vi "VCI Read Board Info.vi"(8 "error in (no error)":errorcluster, 10 "DevIndex":u32, 11 "DevType":u32) -> (0 "error out":errorcluster, 2 "function return":u32, 3 "pInfo":T1)   [LabVIEW 2012, in "ControlCAN.lvlib"]
doc: "unsigned int WINAPI VCI_ReadBoardInfo(unsigned int DevType,unsigned int DevIndex,PVCI_BOARD_INFO pInfo);"
uses:
  ControlCAN.lvlib
  Ginkgo_Driver.dll
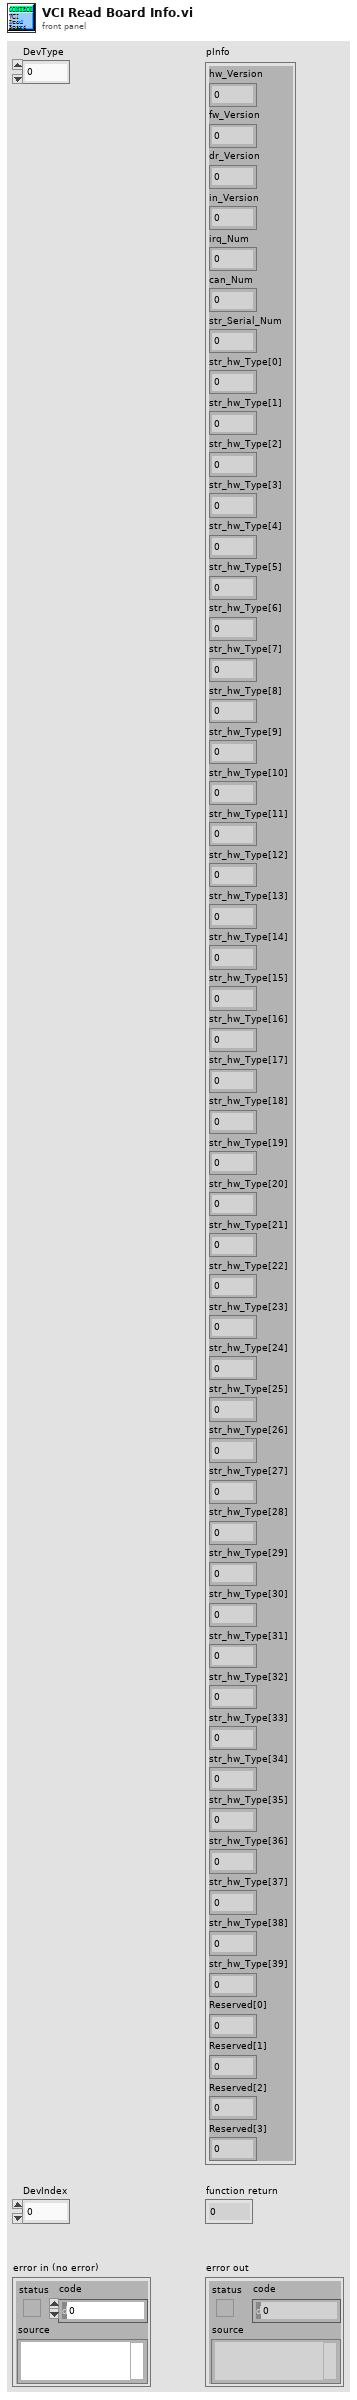
[diagram p1: front panel]
types:
  T1 = cluster{"hw_Version":u16, "fw_Version":u16, "dr_Version":u16, "in_Version":u16, "irq_Num":u16, "can_Num":u8, "str_Serial_Num":u8, "str_hw_Type[0]":u8, "str_hw_Type[1]":u8, "str_hw_Type[2]":u8, "str_hw_Type[3]":u8, "str_hw_Type[4]":u8, "str_hw_Type[5]":u8, "str_hw_Type[6]":u8, "str_hw_Type[7]":u8, "str_hw_Type[8]":u8, "str_hw_Type[9]":u8, "str_hw_Type[10]":u8, "str_hw_Type[11]":u8, "str_hw_Type[12]":u8, "str_hw_Type[13]":u8, "str_hw_Type[14]":u8, "str_hw_Type[15]":u8, "str_hw_Type[16]":u8, "str_hw_Type[17]":u8, "str_hw_Type[18]":u8, "str_hw_Type[19]":u8, "str_hw_Type[20]":u8, "str_hw_Type[21]":u8, "str_hw_Type[22]":u8, "str_hw_Type[23]":u8, "str_hw_Type[24]":u8, "str_hw_Type[25]":u8, "str_hw_Type[26]":u8, "str_hw_Type[27]":u8, "str_hw_Type[28]":u8, "str_hw_Type[29]":u8, "str_hw_Type[30]":u8, "str_hw_Type[31]":u8, "str_hw_Type[32]":u8, "str_hw_Type[33]":u8, "str_hw_Type[34]":u8, "str_hw_Type[35]":u8, "str_hw_Type[36]":u8, "str_hw_Type[37]":u8, "str_hw_Type[38]":u8, "str_hw_Type[39]":u8, "Reserved[0]":u16, "Reserved[1]":u16, "Reserved[2]":u16, "Reserved[3]":u16}
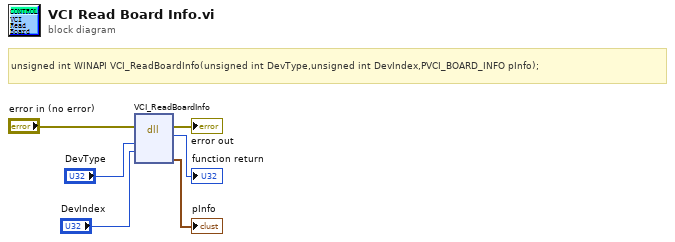
[diagram p0: block diagram]
diagram:
  # "unsigned int WINAPI VCI_ReadBoardInfo(unsigned int DevType,unsigned int DevIndex,PVCI_BOARD_INFO pInfo);"
  n1 = dll-call lib="E:/Project/vt_ginkgo/truck/Ginkgo Driver/vs2010/Ginkgo_USB-I2C_API_v2.0.3.0/lib/labview_32bit/ControlCAN/Ginkgo_Driver.*" fn="VCI_ReadBoardInfo"(error in="error in (no error)", "DevType"="DevType", "DevIndex"="DevIndex") -> (error out=→"error out":errorcluster, →"function return":u32, "pInfo"=→"pInfo":T1)  [unwired: 5 in, 1 out]
